vi "Phasor Convert (tau, f) to (g, s).vi"(1 "Lifetime":dbl[unit], 2 "Phasor Frequency":dbl[unit]) -> (6 "Phasor (g, s)":T1)   [LabVIEW 2021, in "Phasor.lvlib"]
uses:
  Phasor.lvlib
  Phasor (g, s).ctl
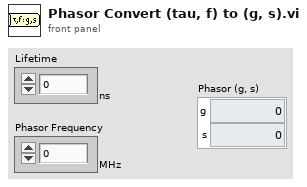
[diagram p1: front panel]
types:
  T1 = typedef "Phasor.lvlib/Phasor (g, s).ctl" = cluster{"g":dbl, "s":dbl}
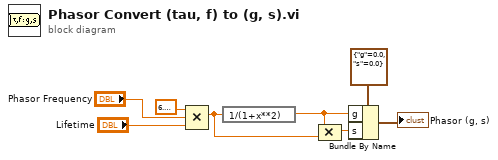
[diagram p0: block diagram]
diagram:
  n1 = Compound Arithmetic op=MULTIPLY(6.283185307179586, "Phasor Frequency", "Lifetime") -> (w1:dbl)
  n2 = expression code="1/(1+x**2)"(w1) -> (w3:dbl)
  n3 = Compound Arithmetic op=MULTIPLY(w3, w1) -> (w2:dbl)
  n4 = Bundle By Name(cluster=T1 {"g"=0.0, "s"=0.0} ("Phasor (g, s)"), "g"=w3, "s"=w2) -> (→"Phasor (g, s)":T1)
